vi "test_libssh2_session_init.vi"() -> ()   [LabVIEW 2017, in "unit_tests.lvlib"]
uses:
  unit_tests.lvlib
  libssh2/libssh2_init_default.vi
  libssh2/libssh2_session_init_ex.vi
  libssh2/libssh2.lvlib
  <vilib>/PNR/Transparent Assertions/Transparent Assertions/Transparent Assertions.lvlib
panel:
  out "error out":errorcluster
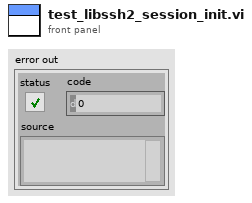
[diagram p1: front panel]
types:
  T1 = typedef "libssh2.lvlib/Session Refnum.ctl" = refnum<k1>
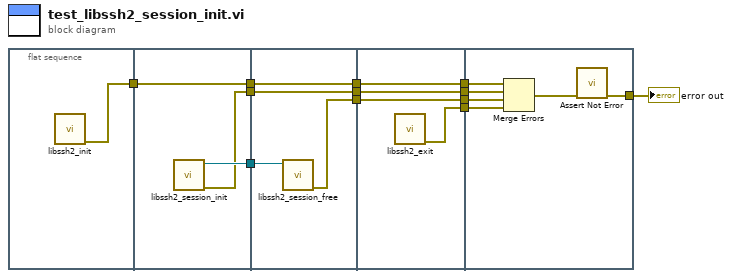
[diagram p0: block diagram]
diagram:
  n1 = flat-sequence {
    tunnel: [w13] -> w8
    tunnel: w8 -> [w16]
    tunnel: [w16] -> w5
    tunnel: [w15] -> w4
    tunnel: [w14] -> w3
    tunnel: w5 -> [w20]
    tunnel: [w20] -> w7
    tunnel: [w19] -> w6
    tunnel: w4 -> [w18]
    tunnel: w3 -> [w17]
    tunnel: [w17] -> w2
    tunnel: w7 -> [w24]
    tunnel: [w24] -> w12
    tunnel: [w23] -> w11
    tunnel: [w22] -> w10
    tunnel: w6 -> [w22]
    tunnel: w2 -> [w21]
    tunnel: [w21] -> w1
    tunnel: w12 -> [w30]
    tunnel: w11 -> [w29]
    tunnel: [w27] -> w9
    tunnel: w10 -> [w26]
    tunnel: w1 -> [w25]
    frame #0 {
      n2 = call-poly "libssh2_init.vi"() -> ("error out"=w13:errorcluster)  [unwired: 11 in]
    }
    frame #1 {
      n3 = call "libssh2_session_init.vi"() -> ("error out"=w14:errorcluster, "session"=w15:T1)  [unwired: 10 in]
    }
    frame #2 {
      n4 = call "libssh2_session_free.vi"("session"=w18) -> ("error out"=w19:errorcluster)  [unwired: 10 in]
    }
    frame #3 {
      n5 = call "libssh2_exit.vi"() -> ("error out"=w23:errorcluster)  [unwired: 11 in]
    }
    frame #4 {
      n6 = Merge Errors(w30, w25, w26, w29) -> (w28:errorcluster)
      n7 = call <vilib>:"Assert Not Error.vi"("error in (no error)"=w28) -> ("error out"=w27:errorcluster)  [unwired: 10 in]
    }
  }
  "error out" <- w9
